vi "start.vi"() -> ()   [LabVIEW 2024]
panel:
  in  "stop":bool
  in  "Duel":bool
  in  "一般模式":bool
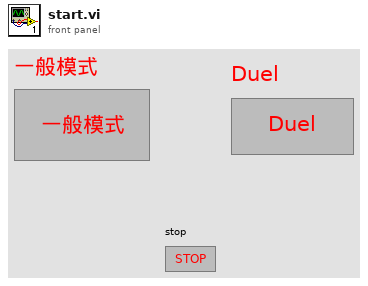
[diagram p1: front panel]
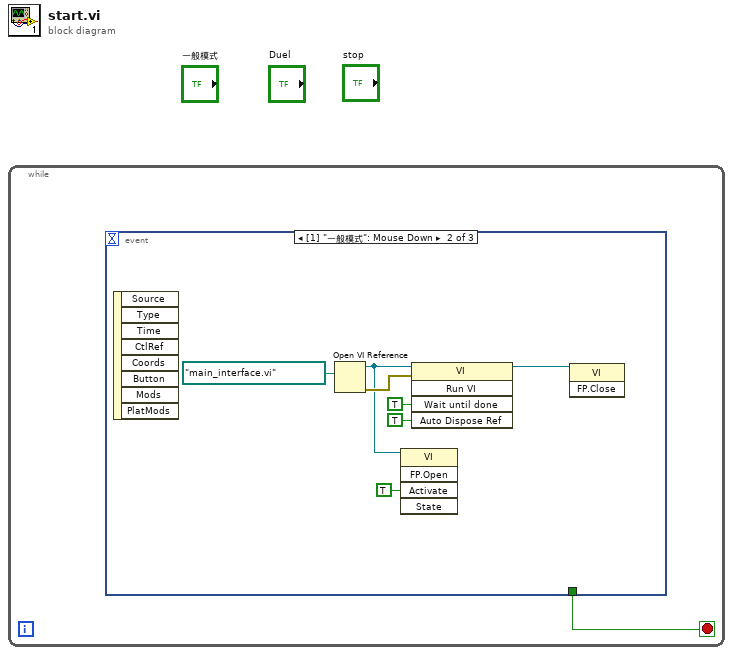
[diagram p0: block diagram]
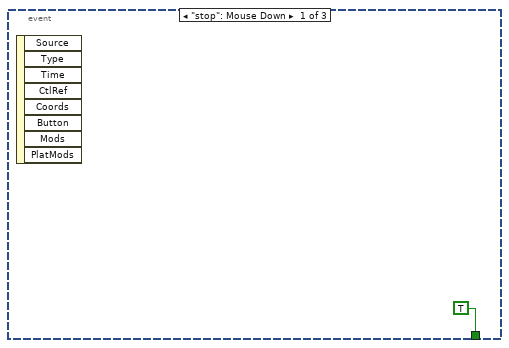
[diagram p2: hidden frame]
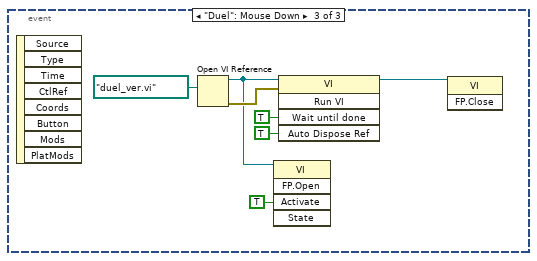
[diagram p3: hidden frame]
diagram:
  n1 = while {
    stop <- w1 stop-if-true
    n2 = event shown="[1] \"一般模式\": Mouse Down" {
      selector: _ -> [_ _ _]
      dyn-events: _ -> [_ _ _]
      timeout: _ -> [_ _ _]
      tunnel: [TRUE _ _] -> w1
      event "stop": Mouse Down {
        n3 = event-data() -> ()  [unwired: 1 in, 8 out]
      }
      event "一般模式": Mouse Down {
        n4 = event-data() -> ()  [unwired: 1 in, 8 out]
        n5 = Open VI Reference(vi path=path "main_interface.vi") -> (vi reference=w5:refnum<vi>, error out=w9:errorcluster)  [unwired: 5 in]
        n6 = invoke class="VI" method="FP.Open"(reference=w5, "Activate"=TRUE ("Activate?")) -> ()  [unwired: 3 in, 5 out]
        n7 = invoke class="VI" method="Run VI"(reference=w5, error in=w9, "Wait until done"=TRUE ("Wait Until Done"), "Auto Dispose Ref"=TRUE ("Auto Dispose Reference")) -> (reference out=w3:refnum<vi>)  [unwired: 1 in, 4 out]
        n8 = invoke class="VI" method="FP.Close"(reference=w3) -> ()  [unwired: 2 in, 3 out]
      }
      event "Duel": Mouse Down {
        n9 = event-data() -> ()  [unwired: 1 in, 8 out]
        n10 = Open VI Reference(vi path=path "duel_ver.vi") -> (vi reference=w11:refnum<vi>, error out=w16:errorcluster)  [unwired: 5 in]
        n11 = invoke class="VI" method="FP.Open"(reference=w11, "Activate"=TRUE ("Activate?")) -> ()  [unwired: 3 in, 5 out]
        n12 = invoke class="VI" method="Run VI"(reference=w11, error in=w16, "Wait until done"=TRUE ("Wait Until Done"), "Auto Dispose Ref"=TRUE ("Auto Dispose Reference")) -> (reference out=w10:refnum<vi>)  [unwired: 1 in, 4 out]
        n13 = invoke class="VI" method="FP.Close"(reference=w10) -> ()  [unwired: 2 in, 3 out]
      }
    }
  }
